vi "1_1_VisualAD_Train_Eval_Test.vi"(0 "NNFE_Paths":T1={"CFG"=path "D:/Ngene/GitHub/deepltk_examples/3_Image_Processing/36_Anomaly_Detection/NNFE/WRN_50_2_2_L3/WRN_50_2_2_BBoneL3.cfg", "BIN"=path "D:/Ngene/GitHub/deepltk_examples/3_Image_Processing/36_Anomaly_Detection/NNFE/WRN_50_2_2_L3/WRN_50_2_2_BBoneL3.bin"}, 1 "Dest. Path":path=path "D:/Ngene/GitHub/deepltk_examples/3_Image_Processing/36_Anomaly_Detection/Models/3OfSpades", 2 "Dataset_Path(Train)":path=path "D:/Ngene/GitHub/deepltk_examples/3_Image_Processing/36_Anomaly_Detection/Dataset/Cards_3OfSpades/train", 3 "Dataset_Path(Validation)":path=path "D:/Ngene/GitHub/deepltk_examples/3_Image_Processing/36_Anomaly_Detection/Dataset/Cards_3OfSpades/test", 4 "Ground_Truth_Folder_Path":path, 5 "error in":errorcluster, 6 "NNFE CFG":T7={"Name"="3OfSpades", "Layer_Selection_By"=enum."Stride", "Feature_Layers"={"[LayerID, PatchSize]"=[{"Layer_ID"=4, "Patch_Size"=3}, {"Layer_ID"=16, "Patch_Size"=5}]}, "Interpolation_Type"=enum."Bi-Linear"}, 7 "Dim_Reduction":T11={"Method"=enum."Rnd_Proj", "Target_Dim"=300, "Seed"=42}, 8 "NNPC_Setup":T2={"Input_Dims"={"C"=3, "H"=320, "W"=272}, "mBatch"=1, "Device"=enum."GPU", "GPU Id"=0}, 9 "CoreSet_Params":T5={"Distance_Metric"=enum."Euclidean", "CoreSet_Size"=10000.0, "Start_idx"=3}) -> (11 "MemBank Size":i32=10000, 13 "dT_Total":dbl=8.530727599999977 format="%.2f", 14 "Model Paths":T1={"CFG"=path "D:/Ngene/GitHub/deepltk_examples/3_Image_Processing/36_Anomaly_Detection/Models/3OfSpades/NNPC_3OfSpades.cfg", "BIN"=path "D:/Ngene/GitHub/deepltk_examples/3_Image_Processing/36_Anomaly_Detection/Models/3OfSpades/NNPC_3OfSpades.bin"}, 15 "Evaluation Metrics":T13={"Evaluation_Metrics(Pixel)"={"Scores(Good)"={"X Values"=[2.1673927682638165, 2.522966259121895, 2.8785397499799728, 3.2341132408380506, 3.589686731696129, 3.945260222554207, 4.300833713412285, 4.656407204270362, 5.011980695128441, 5.367554185986519, 5.723127676844596, 6.078701167702675, 6.434274658560753, 6.78984814941883, 7.145421640276909, 7.500995131134987, 7.856568621993065, 8.212142112851144, 8.567715603709221, 8.923289094567298, 9.278862585425376, 9.634436076283453, 9.990009567141533, 10.345583057999612, 10.70115654885769, 11.056730039715767, 11.412303530573844, 11.767877021431921, 12.12345051229, 12.479024003148078, 12.834597494006157, 13.190170984864235, 13.545744475722312, 13.90131796658039, 14.256891457438469, 14.612464948296546, 14.968038439154626, 15.323611930012703, 15.67918542087078, 16.034758911728858, 16.390332402586935, 16.745905893445013, 17.10147938430309, 17.457052875161168, 17.81262636601925, 18.168199856877326, 18.523773347735403, 18.879346838593484, 19.234920329451562, 19.59049382030964, 19.946067311167717, 20.301640802025794, 20.65721429288387, 21.01278778374195, 21.368361274600026, 21.723934765458107, 22.079508256316185, 22.435081747174262, 22.79065523803234, 23.146228728890417, 23.501802219748498, 23.857375710606576, 24.212949201464653, 24.56852269232273, 24.924096183180808, 25.279669674038885, 25.635243164896963, 25.99081665575504, 26.34639014661312, 26.7019636374712, 27.057537128329276, 27.413110619187353, 27.76868411004543, 28.124257600903512, 28.47983109176159, 28.835404582619667, 29.190978073477744, 29.54655156433582, 29.9021250551939, 30.257698546051977, 30.613272036910054, 30.968845527768135, 31.324419018626212, 31.67999250948429, 32.035566000342364, 32.39113949120044, 32.746712982058526, 33.1022864729166, 33.45785996377468, 33.81343345463276, 34.169006945490835, 34.52458043634891, 34.88015392720699, 35.23572741806507, 35.591300908923145, 35.94687439978122, 36.30244789063931, 36.658021381497385, 37.01359487235546, 37.36916836321354], "Histogram: h(x)"=[1, 13, 52, 84, 115, 188, 266, 742, 1993, 4173, 6263, 6873, 6767, 7084, 7294, 7385, 7892, 8253, 8640, 10003, 11295, 15100, 22306, 35779, 62043, 98920, 135969, 166467, 171557, 159572, 143358, 124535, 97728, 76352, 57016, 39265, 26147, 16432, 10767, 6225, 3406, 1671, 480, 165, 84, 0, 0, 0, 0, 0, 0, 0, 0, 0, 0, 0, 0, 0, 0, 0, 0, 0, 0, 0, 0, 0, 0, 0, 0, 0, 0, 0, 0, 0, 0, 0, 0, 0, 0, 0, 0, 0, 0, 0, 0, 0, 0, 0, 0, 0, 0, 0, 0, 0, 0, 0, 0, 0, 0, 0]}, "Scores(Bad)"={"X Values"=[2.1673927682638165, 2.522966259121895, 2.8785397499799728, 3.2341132408380506, 3.589686731696129, 3.945260222554207, 4.300833713412285, 4.656407204270362, 5.011980695128441, 5.367554185986519, 5.723127676844596, 6.078701167702675, 6.434274658560753, 6.78984814941883, 7.145421640276909, 7.500995131134987, 7.856568621993065, 8.212142112851144, 8.567715603709221, 8.923289094567298, 9.278862585425376, 9.634436076283453, 9.990009567141533, 10.345583057999612, 10.70115654885769, 11.056730039715767, 11.412303530573844, 11.767877021431921, 12.12345051229, 12.479024003148078, 12.834597494006157, 13.190170984864235, 13.545744475722312, 13.90131796658039, 14.256891457438469, 14.612464948296546, 14.968038439154626, 15.323611930012703, 15.67918542087078, 16.034758911728858, 16.390332402586935, 16.745905893445013, 17.10147938430309, 17.457052875161168, 17.81262636601925, 18.168199856877326, 18.523773347735403, 18.879346838593484, 19.234920329451562, 19.59049382030964, 19.946067311167717, 20.301640802025794, 20.65721429288387, 21.01278778374195, 21.368361274600026, 21.723934765458107, 22.079508256316185, 22.435081747174262, 22.79065523803234, 23.146228728890417, 23.501802219748498, 23.857375710606576, 24.212949201464653, 24.56852269232273, 24.924096183180808, 25.279669674038885, 25.635243164896963, 25.99081665575504, 26.34639014661312, 26.7019636374712, 27.057537128329276, 27.413110619187353, 27.76868411004543, 28.124257600903512, 28.47983109176159, 28.835404582619667, 29.190978073477744, 29.54655156433582, 29.9021250551939, 30.257698546051977, 30.613272036910054, 30.968845527768135, 31.324419018626212, 31.67999250948429, 32.035566000342364, 32.39113949120044, 32.746712982058526, 33.1022864729166, 33.45785996377468, 33.81343345463276, 34.169006945490835, 34.52458043634891, 34.88015392720699, 35.23572741806507, 35.591300908923145, 35.94687439978122, 36.30244789063931, 36.658021381497385, 37.01359487235546, 37.36916836321354], "Histogram: h(x)"=[8, 31, 105, 130, 214, 331, 610, 1315, 3212, 6453, 8836, 10903, 11627, 10731, 11893, 12681, 12586, 13151, 14679, 16111, 18152, 22770, 29905, 42923, 63976, 97131, 135040, 170047, 186000, 191189, 185809, 165467, 145942, 127004, 108579, 95369, 82034, 66973, 56446, 48734, 41993, 35860, 33251, 29363, 25936, 23587, 20606, 18581, 16403, 14613, 12756, 11558, 10975, 10578, 9887, 8831, 9074, 8615, 7970, 7376, 6857, 6950, 6755, 6391, 5609, 4681, 3976, 3457, 3231, 2862, 2517, 2294, 2141, 1977, 1864, 1796, 1866, 1798, 1579, 1481, 1246, 1074, 1034, 809, 645, 542, 391, 316, 340, 331, 318, 257, 219, 149, 152, 115, 99, 73, 53, 45]}, "Eval Stats"={"Scores(Good)"={"Min"=2.329183, "Max"=17.973423}, "Scores(Bad)"={"Min"=1.989606, "Max"=37.546955}, "# of Samples(Good)"=1566720, "# of Samples(Bad)"=2611200, "AUROC"=-1.0, "F1_Max"=-1.0, "Thrshld(F1_Max)"=17.973423, "Prec.(F1_Max)"=-1.0, "Recall(F1_Max)"=-1.0, "FPR(F1_Max)"=-1.0, "FNR(F1_Max)"=-1.0}}, "Evaluation_Metrics(Image)"={"Scores(Good)"={"X Values"=[16.63672716140747, 16.8714089012146, 17.10609064102173, 17.34077238082886, 17.575454120635985, 17.810135860443115, 18.044817600250244, 18.279499340057374, 18.514181079864503, 18.74886281967163, 18.98354455947876, 19.218226299285888, 19.452908039093018, 19.687589778900147, 19.922271518707277, 20.156953258514406, 20.391634998321535, 20.62631673812866, 20.86099847793579, 21.09568021774292, 21.33036195755005, 21.565043697357176, 21.799725437164305, 22.034407176971435, 22.269088916778564, 22.503770656585694, 22.738452396392823, 22.973134136199953, 23.207815876007082, 23.44249761581421, 23.677179355621337, 23.911861095428467, 24.146542835235596, 24.381224575042726, 24.615906314849852, 24.85058805465698, 25.08526979446411, 25.31995153427124, 25.55463327407837, 25.7893150138855, 26.02399675369263, 26.258678493499758, 26.493360233306888, 26.728041973114017, 26.962723712921143, 27.197405452728272, 27.4320871925354, 27.666768932342528, 27.901450672149657, 28.136132411956787, 28.370814151763916, 28.605495891571046, 28.840177631378175, 29.074859371185305, 29.309541110992434, 29.544222850799564, 29.77890459060669, 30.01358633041382, 30.24826807022095, 30.482949810028074, 30.717631549835204, 30.952313289642333, 31.186995029449463, 31.421676769256592, 31.656358509063722, 31.89104024887085, 32.12572198867798, 32.36040372848511, 32.59508546829224, 32.82976720809936, 33.06444894790649, 33.29913068771362, 33.53381242752075, 33.76849416732788, 34.00317590713501, 34.23785764694214, 34.47253938674927, 34.7072211265564, 34.94190286636353, 35.17658460617066, 35.411266345977786, 35.645948085784916, 35.880629825592045, 36.115311565399175, 36.349993305206304, 36.584675045013434, 36.819356784820556, 37.054038524627686, 37.288720264434815, 37.523402004241944, 37.758083744049074, 37.9927654838562, 38.22744722366333, 38.462128963470455, 38.696810703277585, 38.931492443084714, 39.166174182891844, 39.40085592269897, 39.6355376625061, 39.87021940231323], "Histogram: h(x)"=[2, 0, 0, 1, 2, 0, 1, 2, 3, 3, 2, 1, 0, 0, 1, 0, 0, 0, 0, 0, 0, 0, 0, 0, 0, 0, 0, 0, 0, 0, 0, 0, 0, 0, 0, 0, 0, 0, 0, 0, 0, 0, 0, 0, 0, 0, 0, 0, 0, 0, 0, 0, 0, 0, 0, 0, 0, 0, 0, 0, 0, 0, 0, 0, 0, 0, 0, 0, 0, 0, 0, 0, 0, 0, 0, 0, 0, 0, 0, 0, 0, 0, 0, 0, 0, 0, 0, 0, 0, 0, 0, 0, 0, 0, 0, 0, 0, 0, 0, 0]}, "Scores(Bad)"={"X Values"=[16.63672716140747, 16.8714089012146, 17.10609064102173, 17.34077238082886, 17.575454120635985, 17.810135860443115, 18.044817600250244, 18.279499340057374, 18.514181079864503, 18.74886281967163, 18.98354455947876, 19.218226299285888, 19.452908039093018, 19.687589778900147, 19.922271518707277, 20.156953258514406, 20.391634998321535, 20.62631673812866, 20.86099847793579, 21.09568021774292, 21.33036195755005, 21.565043697357176, 21.799725437164305, 22.034407176971435, 22.269088916778564, 22.503770656585694, 22.738452396392823, 22.973134136199953, 23.207815876007082, 23.44249761581421, 23.677179355621337, 23.911861095428467, 24.146542835235596, 24.381224575042726, 24.615906314849852, 24.85058805465698, 25.08526979446411, 25.31995153427124, 25.55463327407837, 25.7893150138855, 26.02399675369263, 26.258678493499758, 26.493360233306888, 26.728041973114017, 26.962723712921143, 27.197405452728272, 27.4320871925354, 27.666768932342528, 27.901450672149657, 28.136132411956787, 28.370814151763916, 28.605495891571046, 28.840177631378175, 29.074859371185305, 29.309541110992434, 29.544222850799564, 29.77890459060669, 30.01358633041382, 30.24826807022095, 30.482949810028074, 30.717631549835204, 30.952313289642333, 31.186995029449463, 31.421676769256592, 31.656358509063722, 31.89104024887085, 32.12572198867798, 32.36040372848511, 32.59508546829224, 32.82976720809936, 33.06444894790649, 33.29913068771362, 33.53381242752075, 33.76849416732788, 34.00317590713501, 34.23785764694214, 34.47253938674927, 34.7072211265564, 34.94190286636353, 35.17658460617066, 35.411266345977786, 35.645948085784916, 35.880629825592045, 36.115311565399175, 36.349993305206304, 36.584675045013434, 36.819356784820556, 37.054038524627686, 37.288720264434815, 37.523402004241944, 37.758083744049074, 37.9927654838562, 38.22744722366333, 38.462128963470455, 38.696810703277585, 38.931492443084714, 39.166174182891844, 39.40085592269897, 39.6355376625061, 39.87021940231323], "Histogram: h(x)"=[0, 0, 0, 0, 0, 0, 0, 0, 0, 0, 0, 0, 0, 0, 0, 0, 0, 0, 0, 0, 0, 1, 0, 0, 0, 1, 0, 0, 0, 0, 0, 1, 0, 0, 0, 0, 0, 0, 1, 0, 0, 1, 0, 0, 0, 0, 1, 0, 1, 0, 2, 2, 0, 0, 0, 1, 1, 1, 1, 0, 2, 2, 0, 0, 0, 0, 2, 0, 0, 1, 0, 0, 1, 1, 0, 0, 0, 0, 0, 0, 0, 1, 0, 0, 0, 0, 0, 0, 1, 0, 0, 0, 0, 0, 2, 1, 0, 0, 0, 1]}, "Eval Stats"={"Scores(Good)"={"Min"=16.519386, "Max"=19.817144}, "Scores(Bad)"={"Min"=21.46867, "Max"=39.98756}, "# of Samples(Good)"=18, "# of Samples(Bad)"=30, "AUROC"=1.0904129, "F1_Max"=-1.0, "Thrshld(F1_Max)"=20.642906, "Prec.(F1_Max)"=-1.0, "Recall(F1_Max)"=-1.0, "FPR(F1_Max)"=-1.0, "FNR(F1_Max)"=-1.0}}} {"Evaluation_Metrics(Image)"."Eval Stats"."Recall(F1_Max)" format="%#.5f"; "Evaluation_Metrics(Image)"."Eval Stats"."FPR(F1_Max)" format="%#.5f"; "Evaluation_Metrics(Image)"."Eval Stats"."FNR(F1_Max)" format="%#.5f"; "Evaluation_Metrics(Image)"."Eval Stats"."Prec.(F1_Max)" format="%#.5f"; "Evaluation_Metrics(Image)"."Eval Stats"."F1_Max" format="%#.5f"; "Evaluation_Metrics(Image)"."Eval Stats"."AUROC" format="%#.5f"; "Evaluation_Metrics(Image)"."Eval Stats"."Scores(Bad)"."Min" format="%#_5g"; "Evaluation_Metrics(Image)"."Eval Stats"."Scores(Good)"."Min" format="%#_5g"; "Evaluation_Metrics(Image)"."Eval Stats"."Thrshld(F1_Max)" format="%#_5f"; "Evaluation_Metrics(Pixel)"."Eval Stats"."Recall(F1_Max)" format="%#.5f"; "Evaluation_Metrics(Pixel)"."Eval Stats"."FPR(F1_Max)" format="%#.5f"; "Evaluation_Metrics(Pixel)"."Eval Stats"."FNR(F1_Max)" format="%#.5f"; "Evaluation_Metrics(Pixel)"."Eval Stats"."Prec.(F1_Max)" format="%#.5f"; "Evaluation_Metrics(Pixel)"."Eval Stats"."F1_Max" format="%#.5f"; "Evaluation_Metrics(Pixel)"."Eval Stats"."AUROC" format="%#.5f"; "Evaluation_Metrics(Pixel)"."Eval Stats"."Scores(Bad)"."Min" format="%#_5g"; "Evaluation_Metrics(Pixel)"."Eval Stats"."Scores(Good)"."Min" format="%#_5g"; "Evaluation_Metrics(Pixel)"."Eval Stats"."Thrshld(F1_Max)" format="%#_5f"}, 18 "Dataset Size":i32=20)   [LabVIEW 2020]
uses:
  <vilib>/Ngene/DeepLTK Anomaly Detection Addon/Toolkit/API/Controls/NN_Paths.ctl
  <vilib>/Ngene/DeepLTK Anomaly Detection Addon/Toolkit/API/Controls/NNPC_Setup.ctl
  <vilib>/Ngene/Deep Learning Toolkit/Toolkit/NN_Data/API/NN_Dims(C,H,W).ctl
  <vilib>/Ngene/Deep Learning Toolkit/Toolkit/NN_Network/Controls/NN_Device.ctl
  <vilib>/Ngene/DeepLTK Anomaly Detection Addon/Toolkit/API/Controls/NNPC_Coreset_Params.ctl
  <vilib>/Ngene/DeepLTK Anomaly Detection Addon/Toolkit/API/Controls/Distance_Metric.ctl
  <vilib>/Ngene/DeepLTK Anomaly Detection Addon/Toolkit/API/Controls/NNFE_CFG.ctl
  <vilib>/Ngene/DeepLTK Anomaly Detection Addon/Toolkit/API/Controls/Layer_Selector.ctl
  <vilib>/Ngene/DeepLTK Anomaly Detection Addon/Toolkit/API/Controls/Feature_Layer_Selector.ctl
  <vilib>/Ngene/DeepLTK Anomaly Detection Addon/Toolkit/API/Controls/Interpolation_Selector.ctl
  <vilib>/Ngene/DeepLTK Anomaly Detection Addon/Toolkit/API/Controls/NNPC_Random_Projection_CFG.ctl
  <vilib>/Ngene/DeepLTK Anomaly Detection Addon/Toolkit/API/Controls/Dim_Reduction_Method.ctl
  <vilib>/Ngene/DeepLTK Anomaly Detection Addon/Toolkit/API/Controls/Evaluation_Metrics(Pixel_Image).ctl
  <vilib>/Ngene/DeepLTK Anomaly Detection Addon/Toolkit/API/Controls/Evaluation_Metrics.ctl
  <vilib>/Ngene/DeepLTK Anomaly Detection Addon/Toolkit/API/Controls/Eval_Results.ctl
  <vilib>/Ngene/DeepLTK Anomaly Detection Addon/Toolkit/API/Controls/MinMax.ctl
  subVIs/Dataset_Reader/Controls/Read_Options.ctl
  <vilib>/Ngene/DeepLTK Anomaly Detection Addon/Toolkit/API/Controls/NNPC_PreProcessing_Options.ctl
  <vilib>/Ngene/DeepLTK Anomaly Detection Addon/Toolkit/API/Controls/Crop_CFG.ctl
  <vilib>/Ngene/DeepLTK Anomaly Detection Addon/Toolkit/API/Controls/NNPC_DS_Stats.ctl
  <vilib>/Ngene/DeepLTK Anomaly Detection Addon/Toolkit/API/Controls/Image_Stats_RGB.ctl
  subVIs/Train_Case_Investigation/Controls/Detection_Results.ctl
  <vilib>/Ngene/DeepLTK Anomaly Detection Addon/Toolkit/API/Controls/Feature_Scorer_Params.ctl
  <vilib>/Ngene/DeepLTK Anomaly Detection Addon/Toolkit/API/Controls/Gaussian_Blur.ctl
  <vilib>/Ngene/DeepLTK Anomaly Detection Addon/Toolkit/API/Controls/NNPC_Save_CFG.ctl
  subVIs/Visualizer/Controls/Display_Options.ctl
  subVIs/Visualizer/Controls/ROI_Display_Options.ctl
  subVIs/Visualizer/Controls/Heatmap_Display_Options.ctl
  subVIs/Visualizer/Controls/ColorMap.ctl
  subVIs/Visualizer/Controls/Report_Images_CFG.ctl
  4cc6689b-300a-41eb-b37a-9ba3a5a9262f.vi
  f46c6ce4-2999-47cd-b61f-bf4da423de8f.vi
  <vilib>/Utility/High Resolution Relative Seconds.vi
  <vilib>/Ngene/DeepLTK Anomaly Detection Addon/Toolkit/API/NNPC_Predict/NNPC_Predict(Dataset).vi
  <vilib>/Ngene/DeepLTK Anomaly Detection Addon/Toolkit/API/NNPC_Predict/NNPC_Predict(Single).vi
  <vilib>/Ngene/DeepLTK Anomaly Detection Addon/Toolkit/DeepLTK_Anomaly_Detection_Addon.lvlib
  <vilib>/Ngene/Deep Learning Toolkit/Toolkit/Deep_Learning_Toolkit_by_Ngene.lvlib
  <vilib>/ptbypt/NI_PtbyPt.lvlib
panel:
  out "Last Mouse Position:All Elements":cluster{"X":i32, "Y":i32}={"X"=479, "Y"=53}
  in  "?":enum32{"Train Eval", "Test"}(tab)
  out "dT_Gen_Embed":dbl=0.1599688999999671 format="%.2f"
  out "dT_Coreset":dbl=4.050572499999987 format="%.2f"
  out "Coreset_Max_Distances":sgl[](graph)
  out "dT_NN_Init":dbl=2.456176800000037 format="%.2f"
  out "dT_Read_DS(Train)":dbl=0.1306030000000078 format="%.2f"
  out "dT_Read_DS(Test)":dbl=0.1008939999999825 format="%.2f"
  out "dT_Eval":dbl=0.9340452000000141 format="%.2f"
  out "dT_Predict(DS)":dbl=0.6234673999999814 format="%.2f"
  out "Coreset Max":sgl=72.34939
  out "Feature Size":i32=300
  out "Coreset Min":sgl=12.7185
  in  "Online_Coreset_Params":T5={"Distance_Metric"=enum."Euclidean", "CoreSet_Size"=-1.0, "Start_idx"=3}
  in  "index":i32=17 min=0 max=29
  out "Anomaly Detection Result":T17(plugin-control)
  out "Image_Thrshld (Eval)":sgl=20.6429
  in  "Image_Thrshld(Custom)":sgl=-1.0 format="%_5g"
  out "Pixel_Score(Max)":sgl=29.230766
  out "Image_File_Path":path=path "D:/Ngene/GitHub/deepltk_examples/3_Image_Processing/36_Anomaly_Detection/Dataset/Cards_3OfSpades/test/bad/bad_Cut_Twice_1967.bmp"
  out "Pixel_Thrshld (Eval)":sgl=17.9734
  out "Anomaly?":bool=TRUE
  out "Img_Score":sgl=30.951008
  in  "Pixel_Thrshld(Custom)":sgl=18.1 format="%_5g"
  in  "DS Selector":enum16{"Good", "Bad", "Both"}(ring)=enum."Bad"
  in  "Order":enum16{"Ascending", "Descending", "File"}(ring)
  in  "Heatmap Range":T16={"Min"=17.0, "Max"=19.0} {"Min" format="%#_5g"}
  in  "ROI Color":u32(colorbox)=16717824
  out "dT_Predict":dbl=0.015294491011243817 format="%#_3p"
  in  "Stop":bool
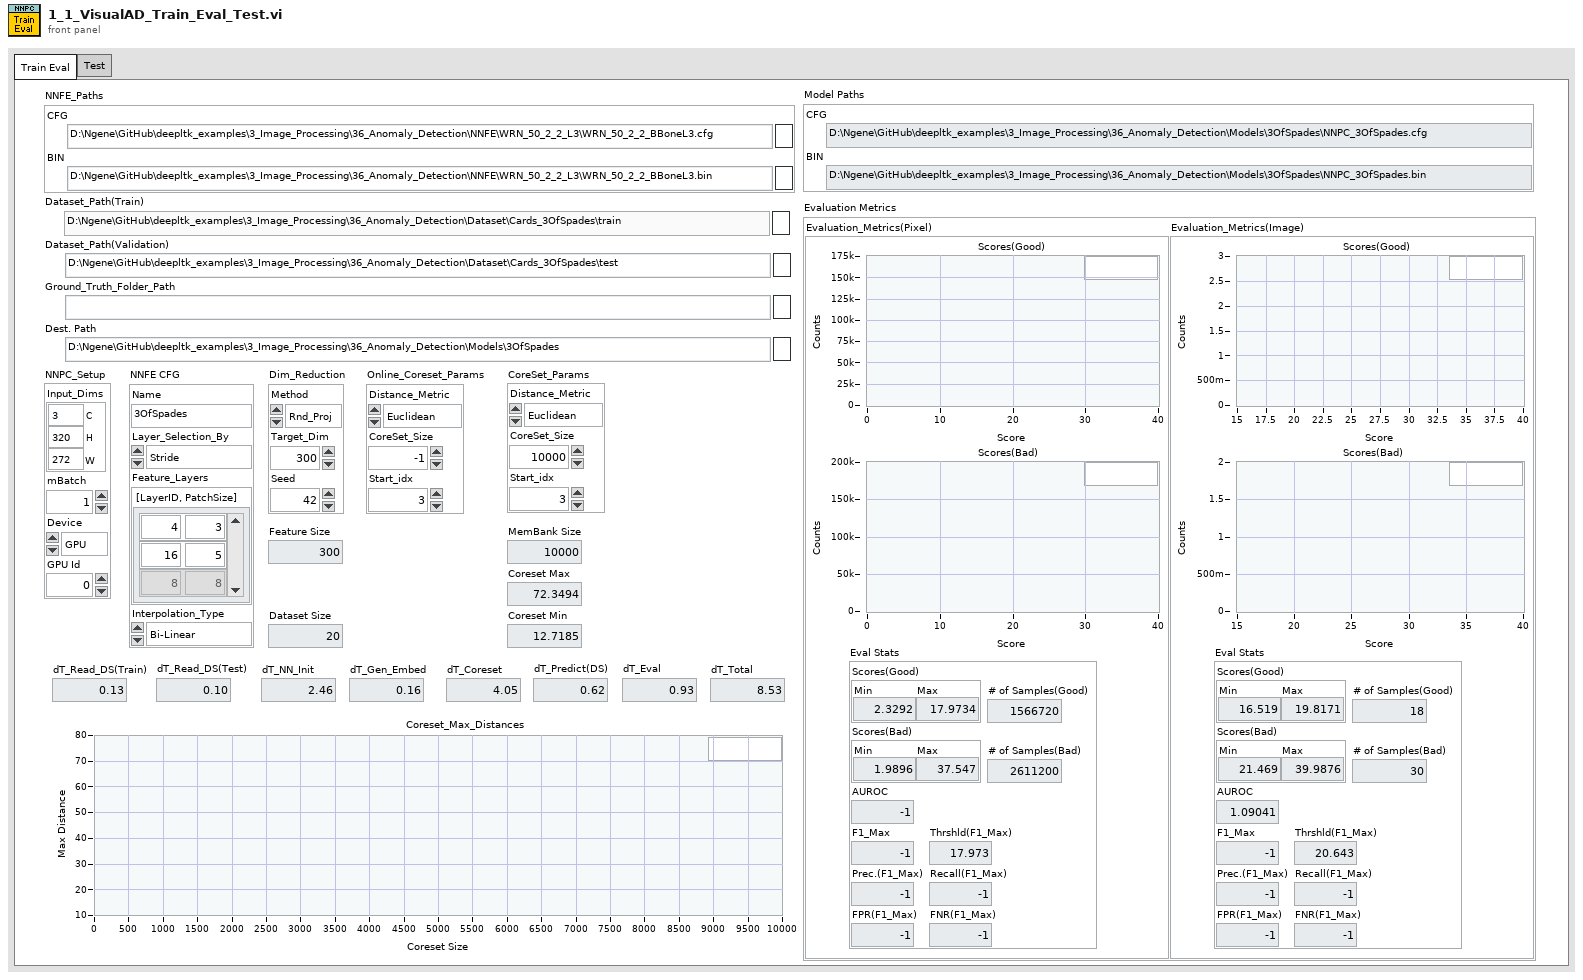
[diagram p1: front panel]
types:
  T1 = typedef "DeepLTK_Anomaly_Detection_Addon.lvlib/NN_Paths.ctl" = cluster{"CFG":path, "BIN":path}
  T2 = typedef "DeepLTK_Anomaly_Detection_Addon.lvlib/NNPC_Setup.ctl" = cluster{"Input_Dims":T3, "mBatch":i32, "Device":T4, "GPU Id":i32}
  T3 = typedef "Deep_Learning_Toolkit_by_Ngene.lvlib/NN_Dims(C,H,W).ctl" = cluster{"C":i32, "H":i32, "W":i32}
  T4 = typedef "Deep_Learning_Toolkit_by_Ngene.lvlib/NN_Device.ctl" = enum16{"CPU", "GPU"}
  T5 = typedef "DeepLTK_Anomaly_Detection_Addon.lvlib/NNPC_Coreset_Params.ctl" = cluster{"Distance_Metric":T6, "CoreSet_Size":sgl, "Start_idx":i32}
  T6 = typedef "DeepLTK_Anomaly_Detection_Addon.lvlib/Distance_Metric.ctl" = enum16{"Euclidean", "Cosine"}
  T7 = typedef "DeepLTK_Anomaly_Detection_Addon.lvlib/NNFE_CFG.ctl" = cluster{"Name":string, "Layer_Selection_By":T8, "Feature_Layers":T9, "Interpolation_Type":T10}
  T8 = typedef "DeepLTK_Anomaly_Detection_Addon.lvlib/Layer_Selector.ctl" = enum16{"Stride", "Layer_Idx"}
  T9 = typedef "DeepLTK_Anomaly_Detection_Addon.lvlib/Feature_Layer_Selector.ctl" = cluster{"[LayerID, PatchSize]":cluster{"Layer_ID":i32, "Patch_Size":i32}[]}
  T10 = typedef "DeepLTK_Anomaly_Detection_Addon.lvlib/Interpolation_Selector.ctl" = enum16{"Nearest", "Bi-Linear"}
  T11 = typedef "DeepLTK_Anomaly_Detection_Addon.lvlib/NNPC_Random_Projection_CFG.ctl" = cluster{"Method":T12, "Target_Dim":i32, "Seed":i32}
  T12 = typedef "DeepLTK_Anomaly_Detection_Addon.lvlib/Dim_Reduction_Method.ctl" = enum16{"None", "Rnd_Proj", "PCA"}
  T13 = typedef "DeepLTK_Anomaly_Detection_Addon.lvlib/Evaluation_Metrics(Pixel_Image).ctl" = cluster{"Evaluation_Metrics(Pixel)":T14, "Evaluation_Metrics(Image)":T14}
  T14 = typedef "DeepLTK_Anomaly_Detection_Addon.lvlib/Evaluation_Metrics.ctl" = cluster{"Scores(Good)":cluster{"X Values":dbl[], "Histogram: h(x)":i32[]}, "Scores(Bad)":cluster{"X Values":dbl[], "Histogram: h(x)":i32[]}, "Eval Stats":T15}
  T15 = typedef "DeepLTK_Anomaly_Detection_Addon.lvlib/Eval_Results.ctl" = cluster{"Scores(Good)":T16, "Scores(Bad)":T16, "# of Samples(Good)":i32, "# of Samples(Bad)":i32, "AUROC":sgl, "F1_Max":sgl, "Thrshld(F1_Max)":sgl, "Prec.(F1_Max)":sgl, "Recall(F1_Max)":sgl, "FPR(F1_Max)":sgl, "FNR(F1_Max)":sgl}
  T16 = typedef "DeepLTK_Anomaly_Detection_Addon.lvlib/MinMax.ctl" = cluster{"Min":sgl, "Max":sgl}
  T17 = typedef "IMAQ Image.ctl" = refnum<image>
  T18 = typedef "DeepLTK_Anomaly_Detection_Addon.lvlib/NNPC_Save_CFG.ctl" = cluster{"Add_TimeStamp_SubFolder":bool, "Append_TimeStamp_to_FileNames":bool}
  T19 = typedef "DeepLTK_Anomaly_Detection_Addon.lvlib/Feature_Scorer_Params.ctl" = cluster{"Nearest_Neighbors":i32, "Calculate Anomaly Map":bool, "Gaussian_Blur":T20}
  T20 = typedef "DeepLTK_Anomaly_Detection_Addon.lvlib/Gaussian_Blur.ctl" = cluster{"Kernel_Size":i32, "Sigma":sgl}
  T21 = typedef "Detection_Results.ctl" = cluster{"Image Score":sgl, "Pixel Score":sgl[][], "File Path":path}
  T22 = typedef "Read_Options.ctl" = cluster{"Read Bads?":bool, "Read GTs?":bool, "Update. DS Stats?":bool}
  T23 = typedef "DeepLTK_Anomaly_Detection_Addon.lvlib/NNPC_PreProcessing_Options.ctl" = cluster{"DS_Name":string, "Input_Dims":T3, "Cropping":T24, "Interpolation Type":u32, "MultiStage_ReSample?":bool, "Dataset_Stats":T25}
  T24 = typedef "DeepLTK_Anomaly_Detection_Addon.lvlib/Crop_CFG.ctl" = cluster{"Left":sgl, "Top":sgl, "Right":sgl, "Bottom":sgl}
  T25 = typedef "DeepLTK_Anomaly_Detection_Addon.lvlib/NNPC_DS_Stats.ctl" = cluster{"means":T26, "stds":T26}
  T26 = typedef "DeepLTK_Anomaly_Detection_Addon.lvlib/Image_Stats_RGB.ctl" = cluster{"R":sgl, "G":sgl, "B":sgl}
  T27 = typedef "Deep_Learning_Toolkit_by_Ngene.lvlib/NN_DataSet(In3D_Out3D).ctl" = cluster{"Dataset_Size":i32, "Dims_In":T3, "Labels":string[], "File Paths":path[], "Outputs Ref.":T28, "Inputs Ref.":variant, "Dims_Out":T3, "Custom_Data":variant}
  T28 = typedef "Deep_Learning_Toolkit_by_Ngene.lvlib/NN_Data_ref(4D_SGL).ctl" = refnum<data-value>
  T29 = typedef "DeepLTK_Anomaly_Detection_Addon.lvlib/NNPC_Instance.ctl" = cluster{"Name":string, "NN":T30, "MemBank_Data":T44}
  T30 = typedef "Deep_Learning_Toolkit_by_Ngene.lvlib/NN.ctl" = cluster{"Name":string, "No of Layers":i32, "mBatch":i32, "Layers":T31[], "Dimty":T32, "Dims_In":T3, "Dims_Out":T3, "Working_Dir":path, "Train?":bool, "Train_Params":T33, "LR_Update_Policy":T36, "Session Data":T38, "Ground_truth":T39, "NNg_hdls":T40, "NN_Device":T4, "GPU Id":i32, "Labels":string[], "Loss_Type":T41, "Loss_Cfg_Prms":variant, "NNG_WS":T42, "DryRun?":bool}
  T31 = typedef "Deep_Learning_Toolkit_by_Ngene.lvlib/NN_Layer_ref.ctl" = refnum<file>
  T32 = typedef "Deep_Learning_Toolkit_by_Ngene.lvlib/NN_In_Out_Dim-ty.ctl" = enum8{"In1D_Out1D", "In3D_Out1D", "In3D_Out3D", "In3D_OutBBox"}
  T33 = typedef "Deep_Learning_Toolkit_by_Ngene.lvlib/NN_Train_Params.ctl" = cluster{"Optimizer":T34, "Beta_1":sgl, "Beta_2":sgl, "Weight Decay(L1)":sgl, "Weight Decay(L2)":sgl, "Data_Sampling":T35}
  T34 = typedef "Deep_Learning_Toolkit_by_Ngene.lvlib/NN_Train_Optimizer.ctl" = enum16{"SGD", "Adam", "Adagrad", "Adadelta", "RMSProp", "Nesterov"}
  T35 = typedef "Deep_Learning_Toolkit_by_Ngene.lvlib/NN_Train_Data_Sampling.ctl" = enum16{"Random", "Sequential"}
  T36 = typedef "Deep_Learning_Toolkit_by_Ngene.lvlib/NN_LR_Policy_Cfg.ctl" = cluster{"Policy_Type":T37, "LR0":dbl, "k":sgl, "WarmUp_Policy":enum16{"Step", "Ramp"}, "WarmUp_Iter":i32, "WarmUp_Ratio":sgl}
  T37 = typedef "Deep_Learning_Toolkit_by_Ngene.lvlib/NN_LR_Policy_Type.ctl" = enum16{"Manual", "Step", "Exp", "1/t"}
  T38 = typedef "Deep_Learning_Toolkit_by_Ngene.lvlib/NN_Train_Session_Data.ctl" = cluster{"Epochs":sgl, "Tot_Iter":i32, "LR":sgl, "LR_iter":i32}
  T39 = typedef "Deep_Learning_Toolkit_by_Ngene.lvlib/NN_Ground_truth.ctl" = cluster{"Y":variant}
  T40 = typedef "Deep_Learning_Toolkit_by_Ngene.lvlib/nng_cuda_handles.ctl" = cluster{"cudnn":u64, "cublas":u64, "stream":u64, "curand":u64}
  T41 = typedef "Deep_Learning_Toolkit_by_Ngene.lvlib/NN_Loss_Type.ctl" = enum16{"None", "MSE", "CrossEntropy", "YOLO_v2", "YOLO_v4"}
  T42 = typedef "Deep_Learning_Toolkit_by_Ngene.lvlib/NNG_WS.ctl" = cluster{"NNG_WS_Mem":T43, "Max_WS_Size":i64}
  T43 = typedef "Deep_Learning_Toolkit_by_Ngene.lvlib/NNg_WS_Mem_DVR.ctl" = refnum<data-value>
  T44 = typedef "DeepLTK_Anomaly_Detection_Addon.lvlib/MemBank_and_Norm_Variants.ctl" = cluster{"MemBank":variant, "MemBank Norm":variant}
  T45 = typedef "imagedata.ctl" = cluster{"image type":i32, "image depth":i32, "image":u8[], "mask":u8[], "colors":u32[], "Rectangle":cluster{"left":i16, "top":i16, "right":i16, "bottom":i16}}
  T46 = typedef "DeepLTK_Anomaly_Detection_Addon.lvlib/NNPC_Evaluation_Results.ctl" = cluster{"Threshold(Image)":sgl, "Threshold(Pixel)":sgl, "Pixel_Range":cluster{"Min":sgl, "Max":sgl}}
  T47 = typedef "Display_Options.ctl" = cluster{"ROI_Options":T48, "Heatmap_Options":T49, "Report_Images_CFG":T51}
  T48 = typedef "ROI_Display_Options.ctl" = cluster{"Color":u32, "Width":u32, "Drawing Mode":enum16{"Frame", "Fill"}}
  T49 = typedef "Heatmap_Display_Options.ctl" = cluster{"ColorMap":T50, "Alpha":sgl, "Heatmap Range":T16}
  T50 = typedef "ColorMap.ctl" = enum16{"Jet", "Perula", "Inferno", "Plasma", "Viridis"}
  T51 = typedef "Report_Images_CFG.ctl" = cluster{"Original Image":bool, "Ground Truth":bool, "HeatMap":bool, "Mask":bool, "Segmentation":bool}
  T52 = typedef "Anomaly_Detection_Results_Imgs.ctl" = cluster{"Image":T17, "Ground Truth":T17, "Predicted Heat Map":T17, "Predicted Mask":T17, "Segmentation":T17}
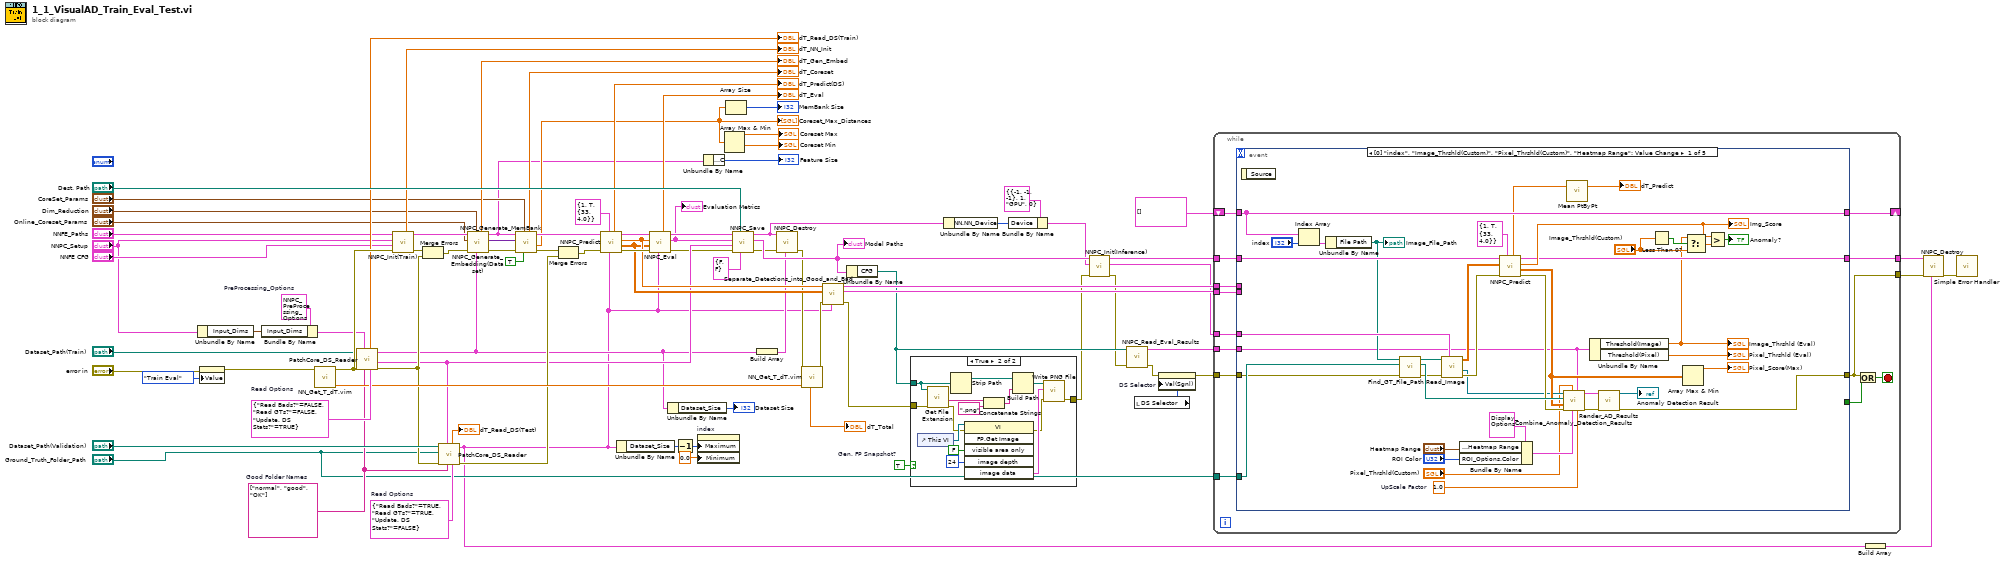
[diagram p0: block diagram]
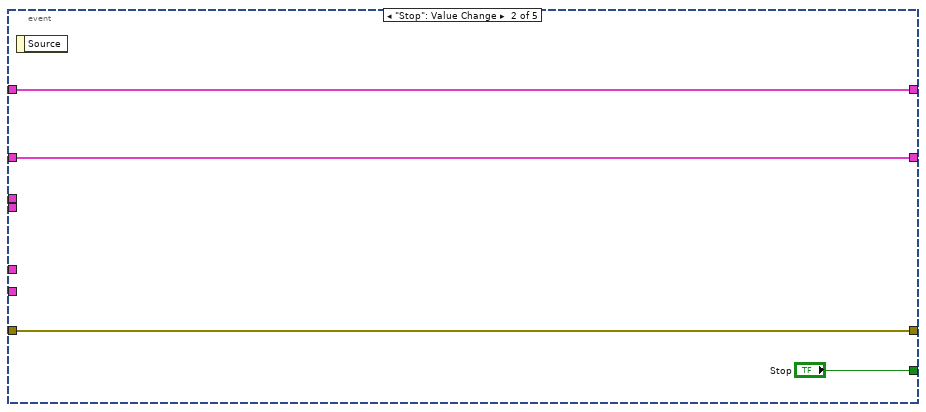
[diagram p2: hidden frame]
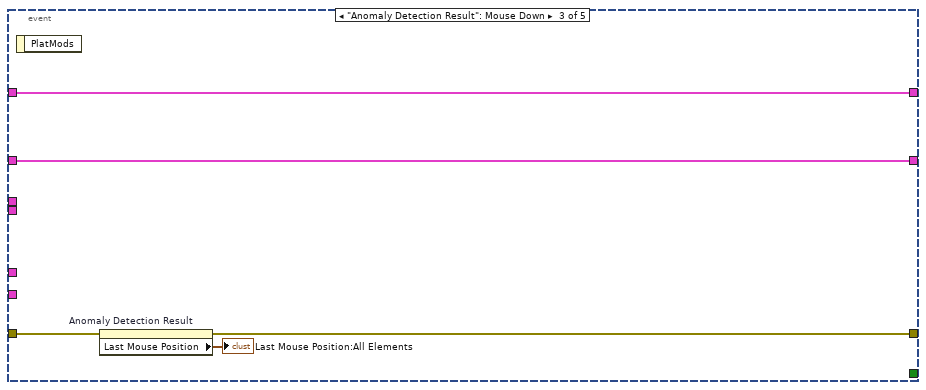
[diagram p3: hidden frame]
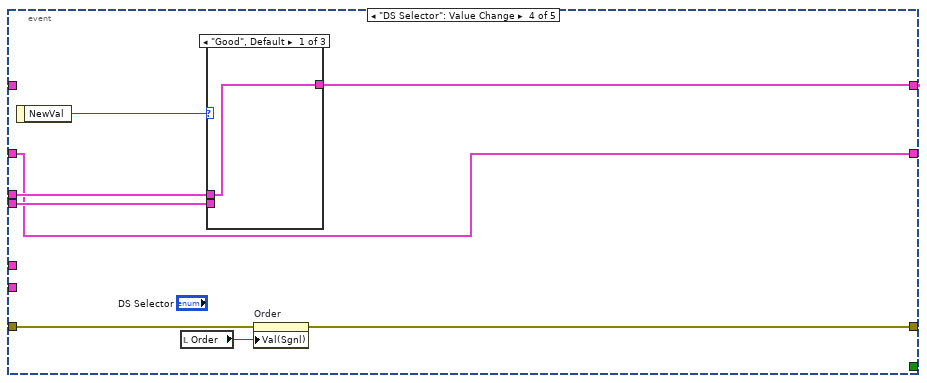
[diagram p4: hidden frame]
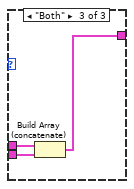
[diagram p6: hidden frame]
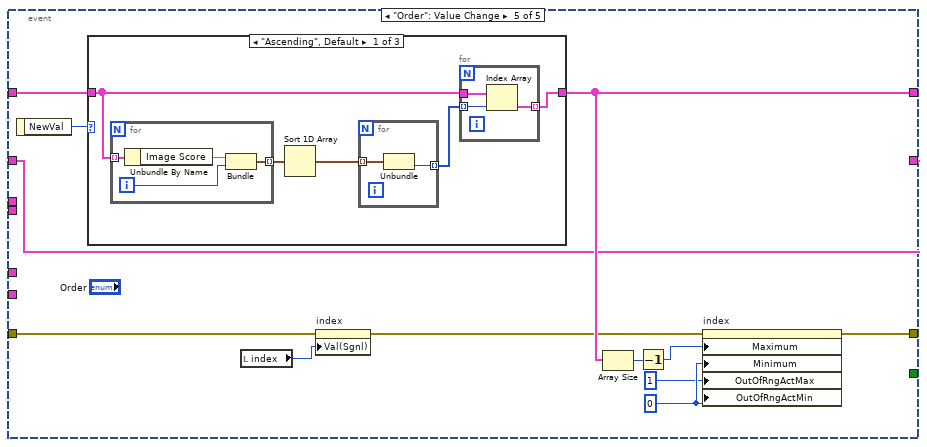
[diagram p7: hidden frame]
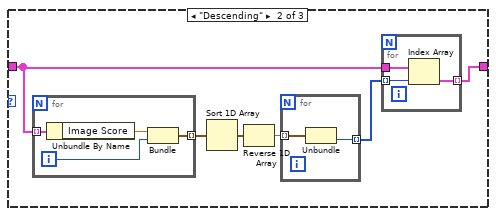
[diagram p8: hidden frame]
diagram:
  w54 = TRUE  # Gen. FP Snapshot?
  w70 = T22 {"Read Bads?"=TRUE, "Read GTs?"=TRUE, "Update. DS Stats?"=FALSE}  # Read Options
  w81 = T23 {"DS_Name"="", "Input_Dims"={"C"=3, "H"=224, "W"=224}, "Cropping"={"Left"=-1.0, "Top"=-1.0, "Right"=-1.0, "Bottom"=-1.0}, "Interpolation Type"=1, "MultiStage_ReSample?"=TRUE, "Dataset_Stats"={"means"={"R"=0.0, "G"=0.0, "B"=0.0}, "stds"={"R"=1.0, "G"=1.0, "B"=1.0}}}  # PreProcessing_Options
  w78 = T22 {"Read Bads?"=FALSE, "Read GTs?"=FALSE, "Update. DS Stats?"=TRUE}  # Read Options
  w60 = string[] ["normal", "good", "OK"]  # Good Folder Names
  n1 = Unbundle By Name("NNPC_Setup") -> ("Input_Dims"=w79:T3)
  n2 = property class="TabCtl (strict)"(error in="error in", "Value"=enum32{"Train Eval", "Test"}."Train Eval") -> (error out=w46:errorcluster)  [unwired: 1 in, 1 out]
  n3 = Bundle By Name(cluster=w81, "Input_Dims"=w79) -> (w40:T23)
  n4 = call "NN_Get_T_dT.vim"("error in"=w46) -> ("T_out"=w75:dbl, "error out"=w89:errorcluster)  [unwired: 6 in, 1 out]
  n5 = call "PatchCore_DS_Reader.vi"("Read Options"=w78, "Good Unique Labels"=w60, "PreProc_Options_in"=w40, "error in"=w89, "Folder Path"="Dataset_Path(Train)") -> ("error out"=w67:errorcluster, "PreProc_Options_out"=w16:T23, "Dataset"=w6:T27, "dT_DS_Reader"=→"dT_Read_DS(Train)":dbl)  [unwired: 3 in]
  n6 = call <vilib>:"NNPC_Init(Train).vi"("error in"=w89, "NNFE_CFG"="NNFE CFG", "NNPC_Setup"="NNPC_Setup", "NNFE_Paths"="NNFE_Paths") -> ("error out"=w85:errorcluster, "NNPC_out"=w84:T29, "dT_Init_Train"=→"dT_NN_Init":dbl)  [unwired: 5 in]
  n7 = Merge Errors(w85, w67) -> (w76:errorcluster)
  n8 = call "PatchCore_DS_Reader.vi"("Read Options"=w70, "Good Unique Labels"=w60, "PreProc_Options_in"=w16, "error in"=w67, "GT Folder Path"="Ground_Truth_Folder_Path", "Folder Path"="Dataset_Path(Validation)") -> ("error out"=w61:errorcluster, "Dataset"=w5:T27, "dT_DS_Reader"=→"dT_Read_DS(Test)":dbl)  [unwired: 2 in, 1 out]
  n9 = call <vilib>:"NNPC_Generate_Embedding(Dataset).vi"("Dataset"=w6, "Dim_Reduction"="Dim_Reduction", "error in"=w76, "Online_Coreset_Params"="Online_Coreset_Params", "NNPC_in"=w84) -> ("error out"=w23:errorcluster, "Feature_Embeddings"=w72:variant, "NNPC_out"=w41:T29, "dT_Embed"=→"dT_Gen_Embed":dbl)  [unwired: 2 in, 1 out]
  n10 = call <vilib>:"NNPC_Generate_MemBank.vi"("Destroy Embeds Afterwards?"=TRUE, "Coreset_Params"="CoreSet_Params", "error in"=w23, "Feature_Embeddings"=w72, "NNPC_in"=w41) -> ("error out"=w55:errorcluster, "Max_Distances"=w43:sgl[], "NNPC_out"=w63:T29, "dT_Coreset"=→"dT_Coreset":dbl)  [unwired: 2 in, 1 out]
  "Coreset_Max_Distances" <- w43
  n11 = Merge Errors(w55, w61) -> (w62:errorcluster)
  n12 = call-poly <vilib>:"NNPC_Predict.vi"("Dataset"=w5, "Feature_Scorer_Params"=T19 {"Nearest_Neighbors"=1, "Calculate Anomaly Map"=TRUE, "Gaussian_Blur"={"Kernel_Size"=33, "Sigma"=4.0}}, "error in"=w62, "NNPC_in"=w63) -> ("error out"=w64:errorcluster, "Anomaly_Maps"=w51:sgl[][][], "Pred_Scores"=w52:sgl[], "NNPC_out"=w59:T29, "dT_Predict"=→"dT_Predict(DS)":dbl)  [unwired: 3 in]
  n13 = Unbundle By Name(w5) -> ("Dataset_Size"=w34:i32)
  n14 = call <vilib>:"NNPC_Eval.vi"("Dataset"=w5, "error in"=w64, "Anomaly_Maps"=w51, "Pred_Scores"=w52, "NNPC_in"=w59) -> ("error out"=w12:errorcluster, "Evaluation_Metrics"=w7:T13, "NNPC_out"=w58:T29, "dT_Eval"=→"dT_Eval":dbl)  [unwired: 3 in]
  "Evaluation Metrics" <- w7
  n15 = Unbundle By Name(w6) -> ("Dataset_Size"=→"Dataset Size":i32)
  n16 = Decrement(x=w34) -> (x-1=w36:i32)
  n17 = property on="index" class="DigNum (strict)"("Maximum"=w36, "Minimum"=0.0 ("Data Entry Limits:Minimum")) -> ()  [unwired: 2 in, 2 out]
  n18 = Unbundle By Name(w41) -> ("NN.Dims_Out.C"=→"Feature Size":i32)
  n19 = Array Max & Min(array=w43) -> (max value=→"Coreset Max":sgl, min value=→"Coreset Min":sgl)  [unwired: 2 out]
  n20 = Array Size(array=w43) -> (size(s)=→"MemBank Size":i32)
  n21 = call <vilib>:"NNPC_Save.vi"("Save_Config"=T18 {"Add_TimeStamp_SubFolder"=FALSE, "Append_TimeStamp_to_FileNames"=FALSE}, "Dst_Folder"="Dest. Path", "error in"=w12, "PreProc_Options_in"=w16, "Evaluation Metrics"=w7, "NNPC_in"=w58) -> ("error out"=w14:errorcluster, "NNPC_Paths"=w37:T1, "NNPC_out"=w30:T29)  [unwired: 3 in]
  "Model Paths" <- w37
  n22 = Build Array(w6) -> (w8:T27[])
  n23 = call <vilib>:"NNPC_Destroy.vi"("Datasets_to_Destroy"=w8, "error in"=w14, "NNPC_in"=w30) -> ("error out"=w11:errorcluster)  [unwired: 8 in]
  n24 = call "NN_Get_T_dT.vim"("T_in"=w75, "error in"=w11) -> ("error out"=w10:errorcluster, "dT"=→"dT_Total":dbl)  [unwired: 5 in, 1 out]
  n25 = call "Separate_Detections_into_Good_and_Bad.vi"("Dataset"=w5, "error in"=w10, "Pixel Scores"=w51, "Image Scores"=w52) -> ("error out"=w9:errorcluster, "Bad Samples"=w48:T21[], "Good Samples"=w47:T21[])  [unwired: 5 in]
  n26 = Unbundle By Name(w37) -> ("CFG"=w39:path)
  n27 = case shown="True" w54 {
    tunnel: w39 -> [_ w94]
    tunnel: [w90 w93] -> w26
    tunnel: w9 -> [w90 w92]
    frame False {
    }
    frame True {
      n28 = control-ref of="This VI"() -> (w104:refnum<vi>)
      n29 = call <vilib>:"Get File Extension.vi"("error in (no error)"=w92, "file"=w94) -> ("error out"=w91:errorcluster, "filename without extension"=w99:string)  [unwired: 5 in, 3 out]
      n30 = Strip Path(path=w94) -> (stripped path=w96:path)  [unwired: 1 out]
      n31 = invoke class="VI" method="FP.Get Image"(reference=w104, error in=w91, "visible area only"=FALSE ("Visible Area Only"), "image depth"=24 ("Image Depth")) -> (error out=w100:errorcluster, "image data"=w101:T45)  [unwired: 2 in, 4 out]
      n32 = Concatenate Strings(w99, ".png" ("string")) -> (w97:string)
      n33 = Build Path(base path=w96, name or relative path=w97) -> (appended path=w95:path)
      n34 = call <vilib>:"Write PNG File.vi"("error in (no error)"=w100, "image data"=w101, "path to PNG file"=w95) -> ("error out"=w93:errorcluster)  [unwired: 7 in, 1 out]
    }
  }
  n35 = Unbundle By Name(w30) -> ("NN.NN_Device"=w28:T4)
  n36 = Bundle By Name(cluster=T2 {"Input_Dims"={"C"=-1, "H"=-1, "W"=-1}, "mBatch"=1, "Device"=enum."GPU", "GPU Id"=0} ("NNPC_Setup"), "Device"=w28) -> (w29:T2)
  n37 = call <vilib>:"NNPC_Init(Inference).vi"("error in"=w26, "NNPC_Setup"=w29, "NNPC_Paths"=w37) -> ("error out"=w25:errorcluster, "PreProc_Options"=w15:T23, "NNPC_out"=w21:T29)  [unwired: 4 in, 2 out]
  n38 = call <vilib>:"NNPC_Read_Eval_Results.vi"("error in (no error)"=w25, "CFG file path"=w39) -> ("error out"=w22:errorcluster, "Evaluation_Results"=w38:T46)  [unwired: 8 in]
  n39 = local read "DS Selector"() -> (w49:enum16{"Good", "Bad", "Both"})
  n40 = property on="DS Selector" class="Enum (strict)"(error in=w22, "Val(Sgnl)"=w49) -> (error out=w31:errorcluster)  [unwired: 1 in, 1 out]
  n41 = while {
    tunnel: "Ground_Truth_Folder_Path" -> [w116]
    tunnel: w47 -> [w115]
    tunnel: w48 -> [w114]
    shift-right: [w113] -> _
    shift-left: T21[] [] ("Bad Samples") -> [w112]
    tunnel: w15 -> [w110]
    tunnel: w38 -> [w109]
    tunnel: w21 -> [w108]
    tunnel: [w107] -> w20
    tunnel: w31 -> [w117]
    tunnel: [w106] -> w19
    stop <- w111 stop-if-true
    n42 = event shown="[0] \"index\", \"Image_Thrshld(Custom)\", \"Pixel_Thrshld(Custom)\", \"Heatmap Range\": Value Change" {
      selector: _ -> [_ _ _ _ _]
      dyn-events: _ -> [_ _ _ _ _]
      timeout: _ -> [_ _ _ _ _]
      tunnel: w117 -> [w150 w157 w164 w168 w182]
      tunnel: [w119 w157 w163 w167 w180] -> w106
      tunnel: w116 -> [w151 _ _ _ _]
      tunnel: w115 -> [_ _ _ w172 _]
      tunnel: w114 -> [_ _ _ w171 _]
      tunnel: [w138 w160 w162 w170 w187] -> w113
      tunnel: w112 -> [w138 w160 w162 _ w189]
      tunnel: w110 -> [w139 _ _ _ _]
      tunnel: w109 -> [w126 _ _ _ _]
      tunnel: w108 -> [w136 w159 w161 w166 w179]
      tunnel: [w137 w159 w161 w166 w179] -> w107
      tunnel: [_ "Stop" _ _ _] -> w105
      event "index", "Image_Thrshld(Custom)", "Pixel_Thrshld(Custom)": Value Change {
        w122 = sgl 1.0  # UpScale Factor
        n43 = event-data() -> ()  [unwired: 1 in, 1 out]
        n44 = Index Array(array=w138, index="index") -> (element=w149:T21)
        n45 = Unbundle By Name(w149) -> ("File Path"=w133:path)
        "Image_File_Path" <- w133
        n46 = call "Find_GT_File_Path.vi"("error in"=w150, "GT Mask Folder Path"=w151, "Image File Path"=w133) -> ("error out"=w146:errorcluster, "GT File Path"=w154:path, "Image File Path out"=w147:path)  [unwired: 5 in, 1 out]
        n47 = call "Read_Image.vi"("PreProcessing_Options"=w139, "error in"=w146, "Img Path"=w147) -> ("error out"=w144:errorcluster, "Image Out(Cropped)"=w131:T17, "Image Out (Preproc)"=w132:sgl[][][])  [unwired: 3 in, 3 out]
        n48 = Bundle By Name(cluster=T47 {"ROI_Options"={"Color"=16717824, "Width"=3, "Drawing Mode"=enum."Frame"}, "Heatmap_Options"={"ColorMap"=enum."Jet", "Alpha"=0.4, "Heatmap Range"={"Min"=0.089999996, "Max"=0.18}}, "Report_Images_CFG"={"Original Image"=TRUE, "Ground Truth"=FALSE, "HeatMap"=TRUE, "Mask"=TRUE, "Segmentation"=TRUE}} ("Display_Options"), "Heatmap_Options.Heatmap Range"="Heatmap Range", "ROI_Options.Color"="ROI Color") -> (w129:T47)
        n49 = call-poly <vilib>:"NNPC_Predict.vi"("Feature_Scorer_Params"=T19 {"Nearest_Neighbors"=1, "Calculate Anomaly Map"=TRUE, "Gaussian_Blur"={"Kernel_Size"=33, "Sigma"=4.0}}, "error in"=w144, "Image_in"=w132, "NNPC_in"=w136) -> ("error out"=w140:errorcluster, "Anomaly_Map"=w142:sgl[][], "Pred_Score"=w141:sgl, "NNPC_out"=w137:T29, "dT_Predict"=w135:dbl)  [unwired: 2 in, 1 out]
        "Img_Score" <- w141
        n50 = call "Combine_Anomaly_Detection_Results.vi"("Relative Resolution"=w122, "Evaluation_Results"=w126, "Display_Options"=w129, "Pixel Anomaly Thrshld"="Pixel_Thrshld(Custom)", "error in"=w140, "Anomaly Map"=w142, "Gt File Path"=w154, "Orig Image In"=w131) -> ("error out"=w120:errorcluster, "Anomaly Detection Results"=w121:T52)  [unwired: 1 in, 1 out]
        n51 = call <vilib>:"Mean PtByPt.vi"("x"=w135) -> ("mean"=→"dT_Predict":dbl)  [unwired: 3 in, 1 out]
        n52 = Unbundle By Name(w126) -> ("Threshold(Image)"=w125:sgl, "Threshold(Pixel)"=→"Pixel_Thrshld (Eval)":sgl)
        "Image_Thrshld (Eval)" <- w125
        n53 = call "Render_AD_Results.vi"("error in"=w120, "Anomaly Detection Rresults"=w121) -> ("error out"=w119:errorcluster, "Anomaly Detection Result"=→"Anomaly Detection Result":T17)  [unwired: 8 in]
        n54 = Less Than 0?(x="Image_Thrshld(Custom)") -> (x < 0?=w156:bool)
        n55 = Array Max & Min(array=w142) -> (max value=→"Pixel_Score(Max)":sgl)  [unwired: 3 out]
        n56 = Select(t=w125, s=w156, f="Image_Thrshld(Custom)") -> (s? t:f=w155:sgl)
        n57 = Greater?(x=w141, y=w155) -> (0:→"Anomaly?":bool)
      }
      event "Stop": Value Change {
        n58 = event-data() -> ()  [unwired: 1 in, 1 out]
      }
      event "Anomaly Detection Result": Mouse Down {
        n59 = event-data() -> ()  [unwired: 1 in, 1 out]
        n60 = property on="Anomaly Detection Result" class="ImageControl"(error in=w164) -> (error out=w163:errorcluster, "Last Mouse Position"=→"Last Mouse Position:All Elements":cluster{"X":i32, "Y":i32})  [unwired: 1 in, 1 out]
      }
      event "DS Selector": Value Change {
        n61 = event-data() -> ("NewVal"=w173:enum16{"Good", "Bad", "Both"})  [unwired: 1 in]
        n62 = local read "Order"() -> (w169:enum16{"Ascending", "Descending", "File"})
        n63 = case shown="\"Good\", Default" w173 {
          tunnel: w172 -> [w174 _ w178]
          tunnel: w171 -> [_ w175 w177]
          tunnel: [w174 w175 w176] -> w170
          frame "Good", Default {
          }
          frame "Bad" {
          }
          frame "Both" {
            n64 = Build Array (concatenate)(w178, w177) -> (w176:T21[])
          }
        }
        n65 = property on="Order" class="Enum (strict)"(error in=w168, "Val(Sgnl)"=w169) -> (error out=w167:errorcluster)  [unwired: 1 in, 1 out]
      }
      event "Order": Value Change {
        w185 = u32 0 ("Data Entry Limits:Minimum")
        n66 = event-data() -> ("NewVal"=w190:enum16{"Ascending", "Descending", "File"})  [unwired: 1 in]
        n67 = case shown="\"Ascending\", Default" w190 {
          tunnel: [w191 w207 w220] -> w187
          tunnel: w189 -> [w193 w206 w220]
          frame "Ascending", Default {
            n68 = for {
              tunnel: w193 -> [w202] mode=indexing
              tunnel: [w201] -> w195 mode=indexing
              i -> [w200]
              n69 = Unbundle By Name(w202) -> ("Image Score"=w199:sgl)
              n70 = Bundle("Image Score"=w199, w200) -> (w201:cluster{"Image Score":sgl, i32})  [unwired: 1 in]
            }
            n71 = Sort 1D Array(array=w195) -> (sorted array=w194:cluster{"Image Score":sgl, i32}[])
            n72 = for {
              tunnel: w194 -> [w204] mode=indexing
              tunnel: [w203] -> w192 mode=indexing
              n73 = Unbundle(w204) -> (w203:i32)  [unwired: 1 out]
            }
            n74 = for {
              tunnel: w193 -> [w198]
              tunnel: w192 -> [w197] mode=indexing
              tunnel: [w196] -> w191 mode=indexing
              n75 = Index Array(array=w198, index=w197) -> (element=w196:T21)
            }
          }
          frame "Descending" {
            n76 = for {
              tunnel: w206 -> [w217] mode=indexing
              tunnel: [w216] -> w208 mode=indexing
              i -> [w215]
              n77 = Unbundle By Name(w217) -> ("Image Score"=w214:sgl)
              n78 = Bundle("Image Score"=w214, w215) -> (w216:cluster{"Image Score":sgl, i32})  [unwired: 1 in]
            }
            n79 = Sort 1D Array(array=w208) -> (sorted array=w209:cluster{"Image Score":sgl, i32}[])
            n80 = Reverse 1D Array(array=w209) -> (reversed array=w205:cluster{"Image Score":sgl, i32}[])
            n81 = for {
              tunnel: w205 -> [w219] mode=indexing
              tunnel: [w218] -> w210 mode=indexing
              n82 = Unbundle(w219) -> (w218:i32)  [unwired: 1 out]
            }
            n83 = for {
              tunnel: w206 -> [w213]
              tunnel: w210 -> [w212] mode=indexing
              tunnel: [w211] -> w207 mode=indexing
              n84 = Index Array(array=w213, index=w212) -> (element=w211:T21)
            }
          }
          frame "File" {
          }
        }
        n85 = local read "index"() -> (w183:i32)
        n86 = property on="index" class="DigNum (strict)"(error in=w182, "Val(Sgnl)"=w183) -> (error out=w181:errorcluster)  [unwired: 1 in, 1 out]
        n87 = Array Size(array=w187) -> (size(s)=w186:i32)
        n88 = Decrement(x=w186) -> (x-1=w188:i32)
        n89 = property on="index" class="DigNum (strict)"(error in=w181, "Maximum"=w188, "Minimum"=w185, "OutOfRngActMax"=u8 1 ("Response to Value Outside Limits:Maximum"), "OutOfRngActMin"=w185) -> (error out=w180:errorcluster)  [unwired: 1 in, 1 out]
      }
    }
    n90 = Or(x=w106, y=w105) -> (x .or. y?=w111:bool)
  }
  n91 = Build Array(w5) -> (w4:T27[])
  n92 = call <vilib>:"NNPC_Destroy.vi"("Datasets_to_Destroy"=w4, "error in"=w19, "NNPC_in"=w20) -> ("error out"=w3:errorcluster)  [unwired: 8 in]
  n93 = call <vilib>:"Simple Error Handler.vi"("error in (no error)"=w3) -> ()  [unwired: 4 in, 5 out]
